vi "CSV Read updated test.vi"() -> ()   [LabVIEW 2016]
uses:
  <vilib>/Utility/file.llb/Read Delimited Spreadsheet (string).vi
panel:
  in  "Test No.":i32(ring) items=["0", "1", "2", "3", "4", "5", "6", "7", "8", "9"]
  in  "Stop Button":bool
  in  "CSV Data":string[][](array[string])
  out "Fuel Cutoff":dbl[unit]
  out "Oxidizer Cutoff":dbl[unit]
  out "Diluent Cutoff":dbl[unit]
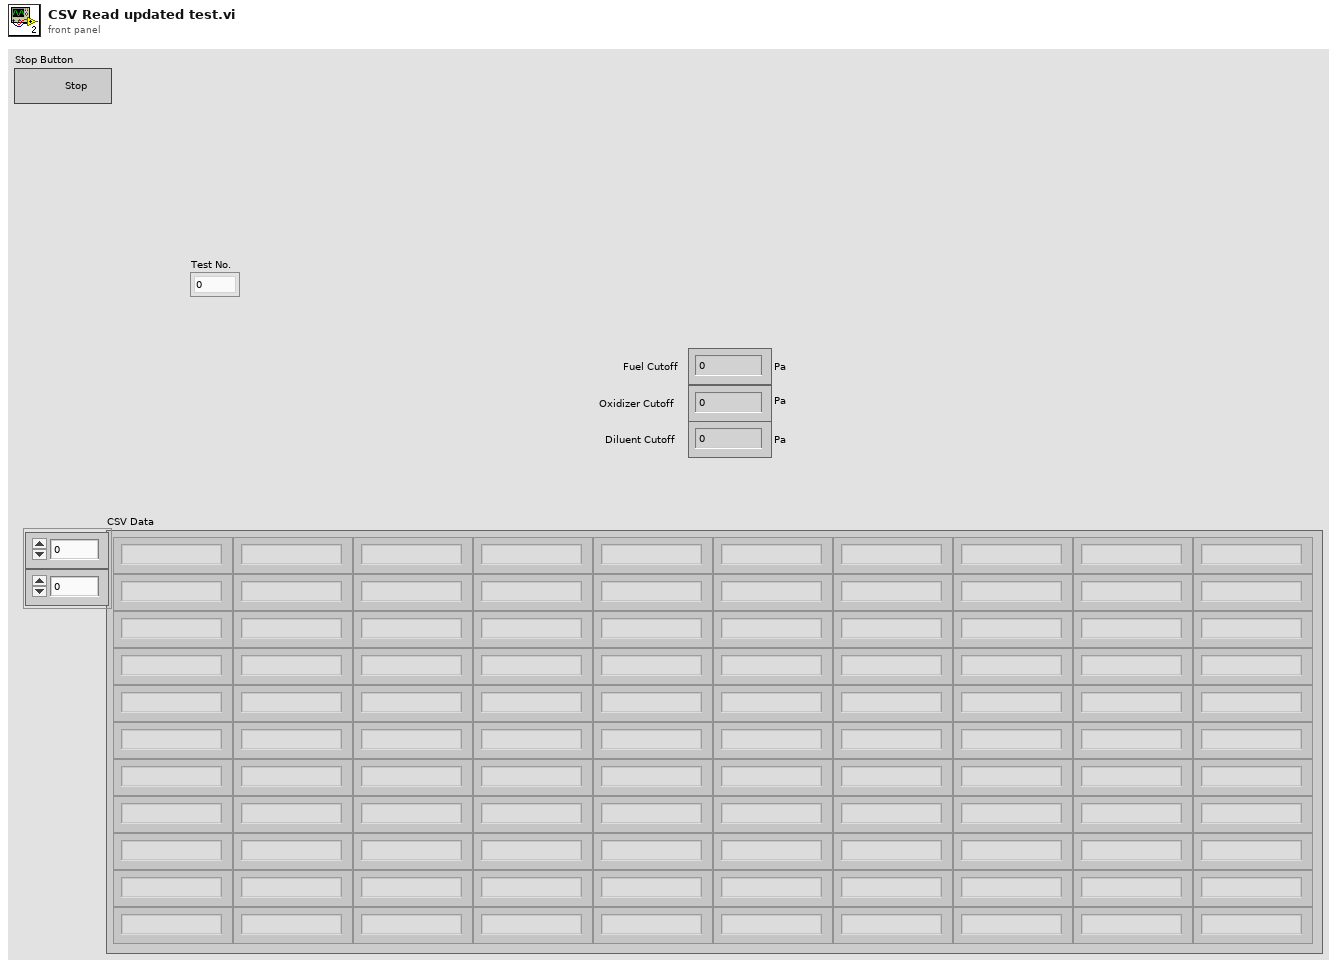
[diagram p1: front panel]
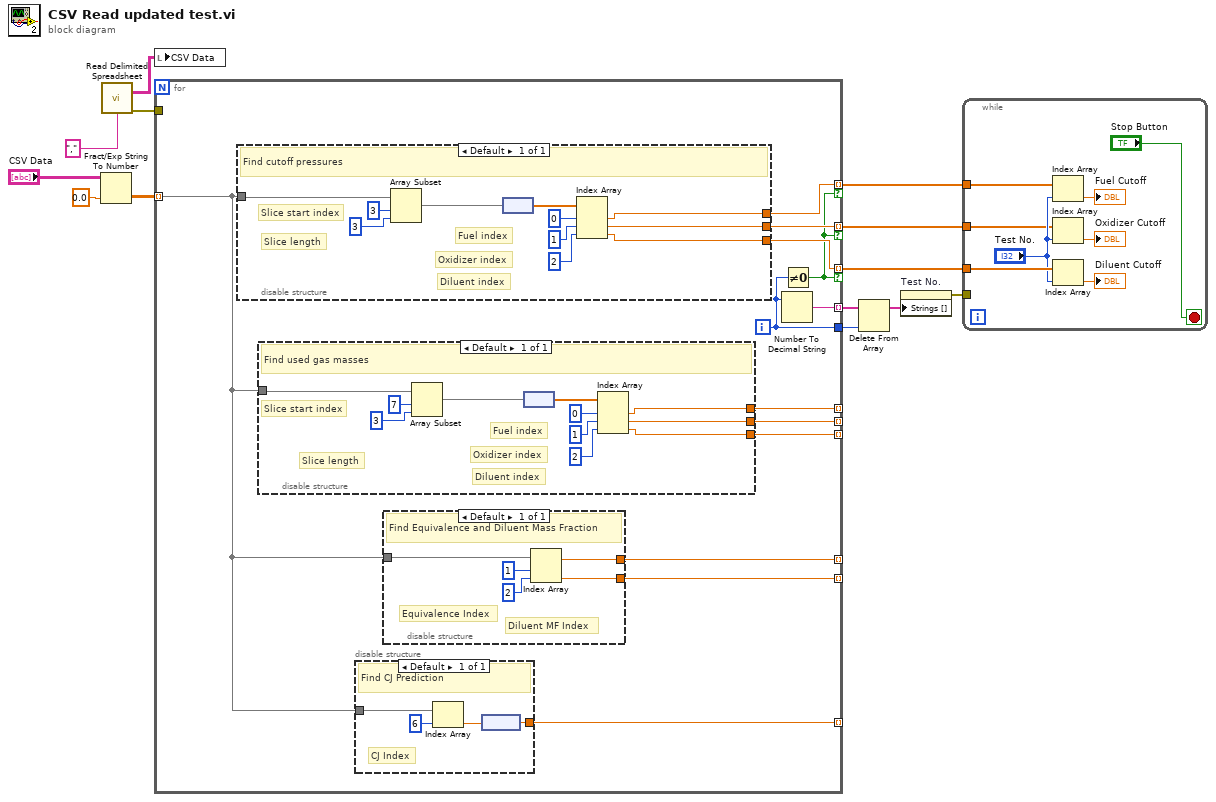
[diagram p0: block diagram]
diagram:
  n1 = Fract/Exp String To Number(string="CSV Data", default (0 dbl)=0.0 ("default (0 I32)")) -> (number=w9:dbl[][])  [unwired: 2 in, 1 out]
  n2 = call-poly <vilib>:"Read Delimited Spreadsheet.vi"("delimiter (\\t)"="," ("delimiter (\\t)")) -> ("all rows"=w13:string[][], "error out"=w6:errorcluster)  [unwired: 9 in, 4 out]
  n3 = local write "CSV Data"(w13) -> ()
  n4 = for {
    tunnel: w9 -> [w26] mode=indexing
    tunnel: [w25] -> w5 mode=indexing if=w15
    tunnel: [w24] -> w4 mode=indexing if=w15
    tunnel: [w23] -> w7 mode=indexing if=w15
    tunnel: [w16] -> w3 mode=indexing
    tunnel: [w22] -> _ mode=indexing
    tunnel: [w21] -> _ mode=indexing
    tunnel: [w20] -> _ mode=indexing
    tunnel: [w19] -> _ mode=indexing
    tunnel: [w18] -> _ mode=indexing
    tunnel: [w17] -> _ mode=indexing
    tunnel: w6 -> [_]
    tunnel: [w14] -> w1
    i -> [w14]
    n5 = disable-structure shown="Default" {
      disable-tunnel: w26 -> [w51]
      disable-tunnel: [w50] -> w25
      disable-tunnel: [w49] -> w24
      disable-tunnel: [w48] -> w23
      frame Enabled {
        # "Slice start index"
        # "Slice length"
        # "Diluent index"
        # "Oxidizer index"
        # "Fuel index"
        # "Find cutoff pressures"
        n6 = Array Subset(array=w51, index=3, length=3) -> (w47:dbl[])
        n7 = node(w47) -> (w53:dbl[unit][])
        n8 = Index Array(array=w53, index #1=0 ("index"), index #2=1 ("index"), index #3=2 ("index")) -> (element #1=w50:dbl[unit], element #2=w49:dbl[unit], element #3=w48:dbl[unit])
      }
    }
    n9 = disable-structure shown="Default" {
      disable-tunnel: w26 -> [w31]
      disable-tunnel: [w30] -> w22
      disable-tunnel: [w29] -> w21
      disable-tunnel: [w28] -> w20
      frame Enabled {
        # "Slice start index"
        # "Slice length"
        # "Diluent index"
        # "Oxidizer index"
        # "Fuel index"
        # "Find used gas masses"
        n10 = Array Subset(array=w31, index=7, length=3) -> (w27:dbl[])
        n11 = node(w27) -> (w32:dbl[unit][])
        n12 = Index Array(array=w32, index #1=0 ("index"), index #2=1 ("index"), index #3=2 ("index")) -> (element #1=w28:dbl[unit], element #2=w29:dbl[unit], element #3=w30:dbl[unit])
      }
    }
    n13 = disable-structure shown="Default" {
      disable-tunnel: w26 -> [w45]
      disable-tunnel: [w43] -> w19
      frame Enabled {
        # "CJ Index"
        # "Find CJ Prediction"
        n14 = Index Array(array=w45, index=6) -> (element=w44:dbl)
        n15 = node(w44) -> (w43:dbl[unit])
      }
    }
    n16 = disable-structure shown="Default" {
      disable-tunnel: w26 -> [w40]
      disable-tunnel: [w39] -> w18
      disable-tunnel: [w38] -> w17
      frame Enabled {
        # "Diluent MF Index"
        # "Equivalence Index"
        # "Find Equivalence and Diluent Mass Fraction"
        n17 = Index Array(array=w40, index #1=1 ("index"), index #2=2 ("index")) -> (element #1=w39:dbl, element #2=w38:dbl)
      }
    }
    n18 = Number To Decimal String(number=w14) -> (decimal integer string=w16:string)  [unwired: 1 in]
    n19 = Not Equal To 0?(x=w14) -> (x != 0?=w15:bool)
  }
  n20 = Delete From Array(array=w3, index=w1) -> (array with subset deleted=w2:string[])  [unwired: 1 in, 1 out]
  n21 = property on="Test No." class="Ring (strict)"("Strings []"=w2) -> (error out=w8:errorcluster)  [unwired: 2 in, 1 out]
  n22 = while {
    tunnel: w8 -> [_]
    tunnel: w7 -> [w64]
    tunnel: w5 -> [w59]
    tunnel: w4 -> [w58]
    stop <- "Stop Button" stop-if-true
    n23 = Index Array(array=w59, index="Test No.") -> (element=→"Fuel Cutoff":dbl[unit])
    n24 = Index Array(array=w58, index="Test No.") -> (element=→"Oxidizer Cutoff":dbl[unit])
    n25 = Index Array(array=w64, index="Test No.") -> (element=→"Diluent Cutoff":dbl[unit])
  }
